vi "Spreadsheet file method.vi"(4 "Flush interval (s)":dbl=60.0 format="%.2f", 5 "File command":T1=enum."Open", 6 "error in (no error)":errorcluster, 7 "1D string":string[](array[string]), 8 "1D num":dbl[](array[numeric]) format="%.2f") -> (0 "error out":errorcluster, 1 "Valid File":bool, 2 "path":path)   [LabVIEW 2010]
uses:
  file command.ctl
panel:
  out "appended path":path
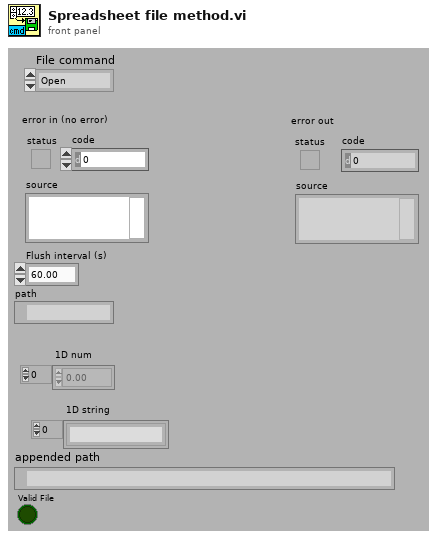
[diagram p1: front panel]
types:
  T1 = typedef "file command.ctl" = enum16{"Open Default", "Open", "Write  num ", "Write text", "Write comment", "Read num", "Read text", "Close"}
  T2 = enum16{"open", "open or create", "create or replace", "create", "open (read only)"}
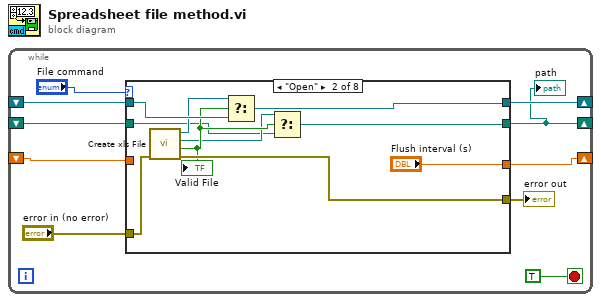
[diagram p0: block diagram]
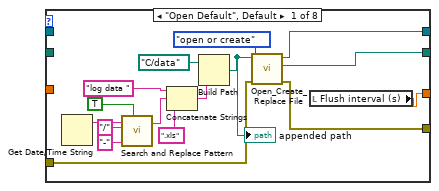
[diagram p2: hidden frame]
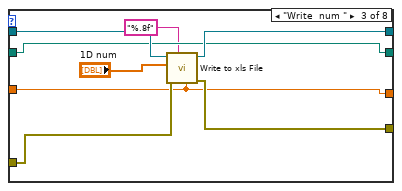
[diagram p3: hidden frame]
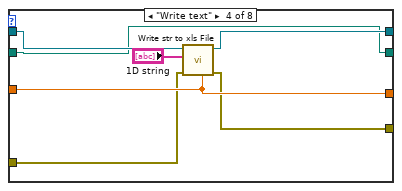
[diagram p4: hidden frame]
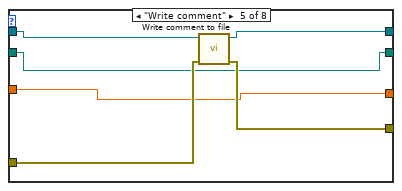
[diagram p5: hidden frame]
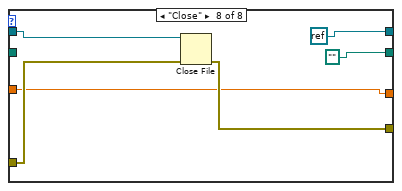
[diagram p8: hidden frame]
diagram:
  n1 = while {
    shift-right: [w7] -> _
    shift-left: _ -> [w6]
    shift-right: [w5] -> _
    shift-left: _ -> [w4]
    shift-right: [w1] -> _
    shift-left: _ -> [w2]
    stop <- TRUE stop-if-true
    n2 = case shown="\"Open\"" "File command" {
      tunnel: [w19 w36 w41 w47 w55 w59 w63 w68] -> w9
      tunnel: "error in (no error)" -> [w23 w35 w42 w48 w56 w59 w63 w69]
      tunnel: [w25 w32 w43 w50 w53 w61 w65 refnum<k0> refnum] -> w7
      tunnel: w6 -> [_ w34 w44 w51 w57 w61 w65 w71]
      tunnel: [w11 "Flush interval (s)" w40 w49 w54 w60 w64 w67] -> w5
      tunnel: w4 -> [_ _ w40 w49 w54 w60 w64 w67]
      tunnel: [w24 w27 w38 w45 w52 w58 w62 path ""] -> w1
      tunnel: w2 -> [_ w28 w38 w45 w52 w58 w62 _]
      frame "Open Default", Default {
        n3 = Get Date/Time String() -> (date string=w18:string)  [unwired: 3 in, 1 out]
        n4 = call <vilib>:"Search and Replace Pattern.vi"("string"=w18, "regular expression (\"\")"="/" ("regular expression (\"\")"), "replace string (\"\")"="-" ("replace string (\"\")"), "replace all? (F)"=TRUE) -> ("result string"=w15:string)  [unwired: 1 in, 1 out]
        n5 = Concatenate Strings("log data " ("name or relative path"), w15, ".xls" ("string")) -> (w20:string)
        n6 = Build Path(base path=path "C:/data", name or relative path=w20) -> (appended path=w26:path)
        "appended path" <- w26
        n7 = call <vilib>:"Open_Create_Replace File.vi"("error in (no error)"=w23, "function (open:0)"=T2."open or create", "file path"=w26) -> ("error out"=w19:errorcluster, "new file path"=w24:path, "refnum"=w25:refnum<file>)  [unwired: 5 in, 1 out]
        n8 = local read "Flush interval (s)"() -> (w11:dbl)
      }
      frame "Open" {
        n9 = call "Create xls File.vi"("error in"=w35) -> ("error out"=w36:errorcluster, "Valid File"=w30:bool, "path"=w29:path, "refnum"=w33:refnum<file>)  [unwired: 3 in]
        "Valid File" <- w30
        n10 = Select(t=w33, s=w30, f=w34) -> (s? t:f=w32:refnum<file>)
        n11 = Select(t=w29, s=w30, f=w28) -> (s? t:f=w27:path)
      }
      frame "Write  num " {
        n12 = call "Write to xls File.vi"("Flush interval (s)"=w40, "format (%.3f)"="%.8f", "error in (no error)"=w42, "1D data"="1D num", "refnum"=w44) -> ("error out"=w41:errorcluster, "dup refnum"=w43:refnum<file>)  [unwired: 5 in]
      }
      frame "Write text" {
        n13 = call "Write str to xls File.vi"("Flush interval (s)"=w49, "error in (no error)"=w48, "1D data"="1D string", "refnum"=w51) -> ("error out"=w47:errorcluster, "dup refnum"=w50:refnum<file>)  [unwired: 6 in]
      }
      frame "Write comment" {
        n14 = call "Write comment to file.vi"("error in (no error)"=w56, "refnum"=w57) -> ("error out"=w55:errorcluster, "dup refnum"=w53:refnum<file>)  [unwired: 6 in]
      }
      frame "Read num" {
      }
      frame "Read text" {
      }
      frame "Close" {
        n15 = Close File(refnum=w71, error in=w69) -> (error out=w68:errorcluster)  [unwired: 1 out]
      }
    }
    "error out" <- w9
    "path" <- w1
  }
